vi "Highlight Row for VI Analyzer.vi"(6 "File Index":i32, 8 "error in":errorcluster, 10 "Review File":string, 11 "Peer Review":refnum<class "Peer Review.lvclass">) -> (0 "error out":errorcluster)   [LabVIEW 2020, in "Peer Review.lvclass"]
uses:
  Peer Review.lvclass
  <vilib>/Utility/miscctls.llb/LVRowAndColumnUnsignedTypeDef.ctl
  Peer Review.lvclass/Peer Review.ctl
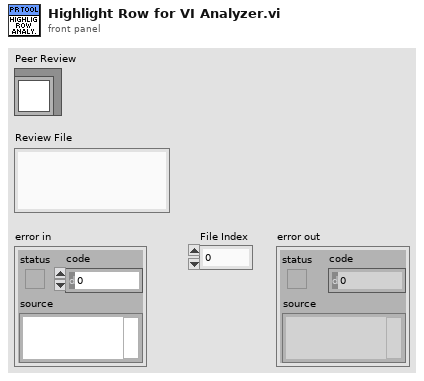
[diagram p1: front panel]
types:
  T1 = typedef "LVRowAndColumnUnsignedTypeDef.ctl" = cluster{"Row":u32, "Column":u32}
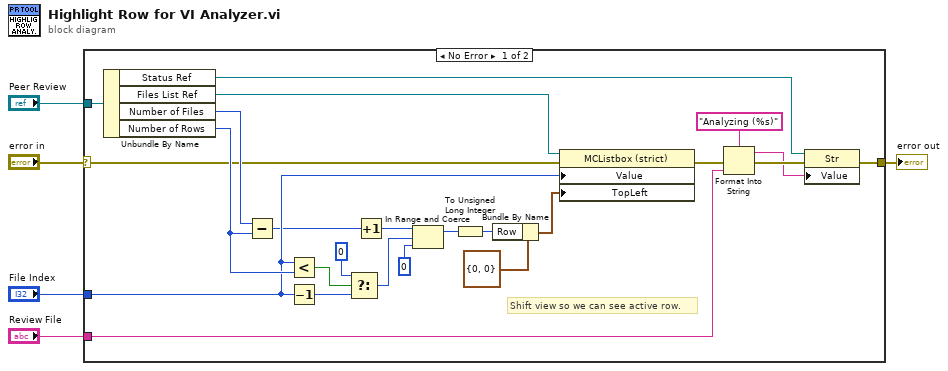
[diagram p0: block diagram]
diagram:
  n1 = case shown="No Error" "error in" {
    selector: "error in" -> [w6 w30]
    tunnel: [w24 w30] -> w4
    tunnel: "Peer Review" -> [w27 _]
    tunnel: "Review File" -> [w25 _]
    tunnel: "File Index" -> [w23 _]
    frame No Error {
      # "Shift view so we can see active row."
      n2 = Unbundle By Name(w27) -> ("Status Ref"=w26:refnum<vi>, "Files List Ref"=w28:refnum<vi>, "Number of Files"=w22:i32, "Number of Rows"=w29:i32)
      n3 = Subtract(x=w22, y=w29) -> (x-y=w20:i32)
      n4 = Less?(x=w23, y=w29) -> (x < y?=w18:bool)
      n5 = Decrement(x=w23) -> (x-1=w17:i32)
      n6 = Select(t=0 ("lower limit"), s=w18, f=w17) -> (s? t:f=w19:i32)
      n7 = Increment(x=w20) -> (x+1=w21:i32)
      n8 = In Range and Coerce(upper limit=w21, x=w19, lower limit=0) -> (coerced(x)=w12:i32)  [unwired: 1 out]
      n9 = To Unsigned Long Integer(number=w12) -> (unsigned 32bit integer=w11:u32)
      n10 = Bundle By Name(cluster=T1 {"Row"=0, "Column"=0} ("Top Left Visible Cell"), "Row"=w11) -> (w16:T1)
      n11 = property class="MCListbox (strict)"(reference=w28, error in=w6, "Value"=w23, "TopLeft"=w16) -> (error out=w9:errorcluster)  [unwired: 1 out]
      n12 = Format Into String(format string="Analyzing (%s)", error in=w9, w25) -> (resulting string=w7:string, error out=w8:errorcluster)  [unwired: 1 in]
      n13 = property class="Str"(reference=w26, error in=w8, "Value"=w7) -> (error out=w24:errorcluster)  [unwired: 1 out]
    }
    frame Error {
    }
  }
  "error out" <- w4
